vi "ABB enter motor data2.vi"(9 "Efficiency Standard":u16(ring) items=["IEC", "NEMA"], 10 "Motor Type":u16(ring) items=["Wound Induction Motor", "Induction Motor", "Synchronous Motor", "Synchronous Generator"], 11 "Efficiency Units":u16(ring) items=["METRIC", "IMPERIAL", "", "", ""]) -> (3 "entered data":string[][](array[string]))   [LabVIEW 2017]
uses:
  ABB global.vi
panel:
  in  "Specified  winding temp rise.":cluster{"Stator":dbl, "Rotor":dbl}
  out "length":i32
  in  "Explosion protection":T1 {"Gas Groups" items=["IIA", "IIB", "IIC"]; "Temp. class" items=["T3", "T2", "T1", "", ""]; "Type" items=["Exd", "EXp", "EXe", "EXn", ""]}
  in  "Synchronous Motor":T2
  in  "Specified Bearing Vibration (mm/Sec rms)":cluster{"Vibration ":dbl}={"Vibration "=1.8}
  in  "Comments":string
  in  "Vibration":T3={"Vibration(mm/sec rms)"=[[0.0, 0.0, 0.0], [0.0, 0.0, 0.0]], "Vibration µm (p-p)"=[[0.0, 0.0, 0.0], [0.0, 0.0, 0.0]], "Shaft vibration µm (p-p)"=[], "Comments"="", "Shaft Vibration"=FALSE, "DE\n\nNDE"="", "String"=""} {"Shaft vibration µm (p-p)" format="%#.2f"; "Vibration µm (p-p)" format="%#.2g"; "Vibration(mm/sec rms)" format="%#.2f"}
  in  "Axial position":T4
  in  "Exit":bool
  # "Enter Motor data 2"
  # "D"
  # "NDE"
  # "Magnetic center(mm)"
  # "-"
  # "-"
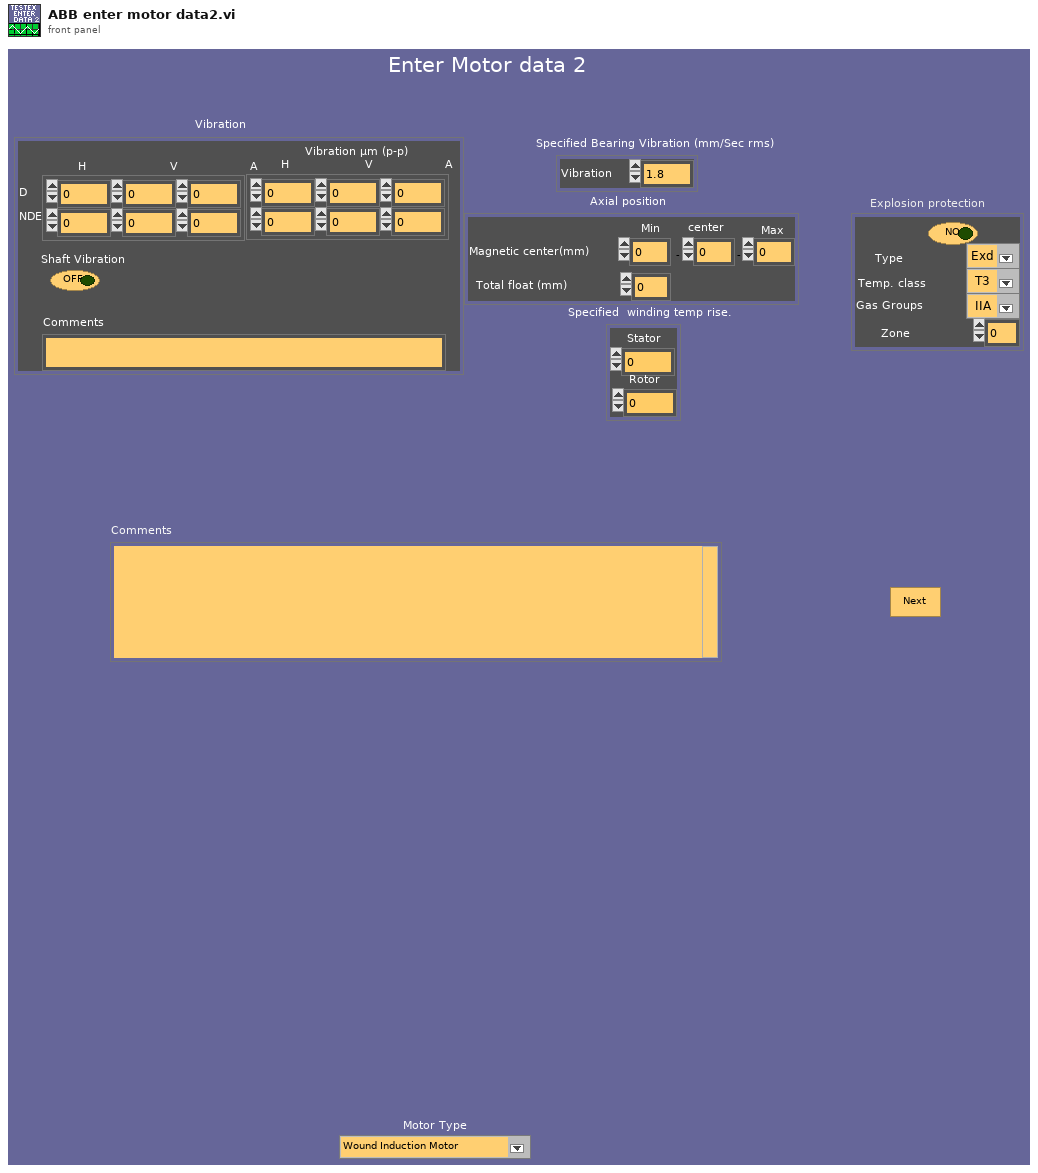
[diagram p1: front panel]
types:
  T1 = cluster{"Explosion protection":bool, "Zone":i32, "Type":u16, "Temp. class":u16, "Gas Groups":u16}
  T2 = cluster{"DC Excitation Amps":dbl, "DC Excitation Volts":dbl}
  T3 = cluster{"Vibration(mm/sec rms)":dbl[][], "Vibration µm (p-p)":dbl[][], "Shaft vibration µm (p-p)":dbl[][], "Comments":string, "Shaft Vibration":bool, "DE\n\nNDE":string, "String":string}
  T4 = cluster{"Min":dbl, " center":dbl, "Max":dbl, "Total float (mm)":dbl}
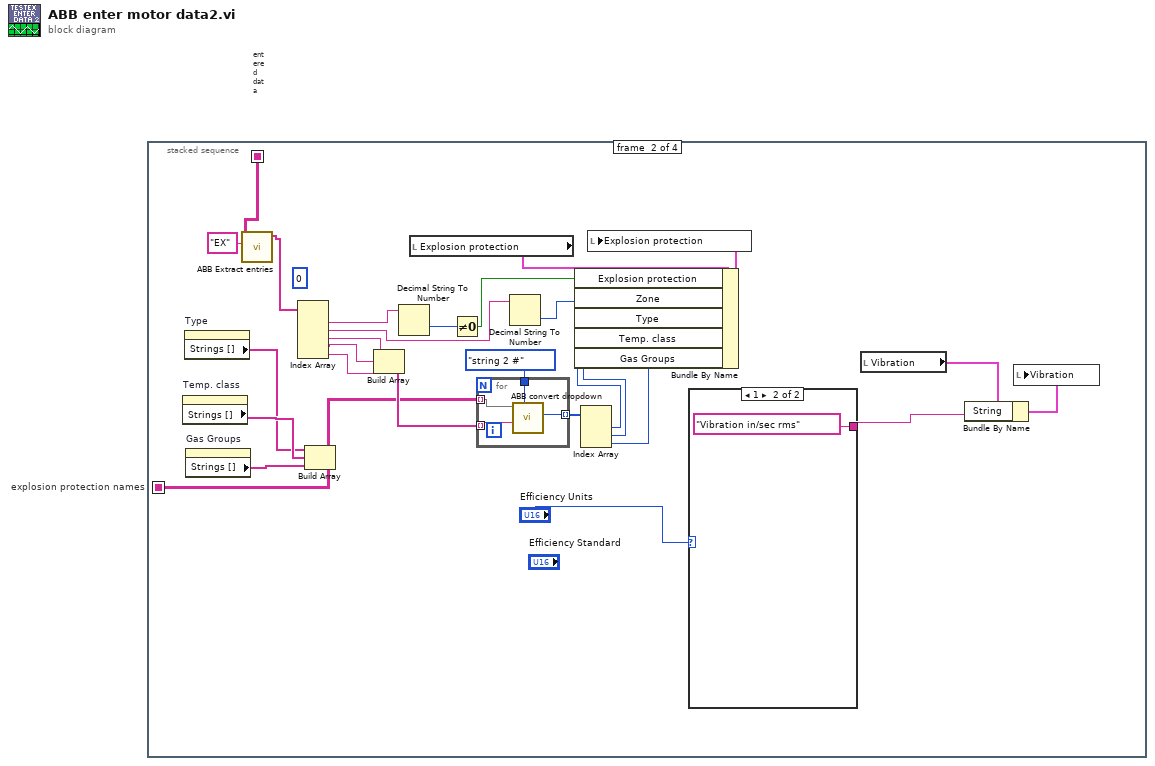
[diagram p0: block diagram]
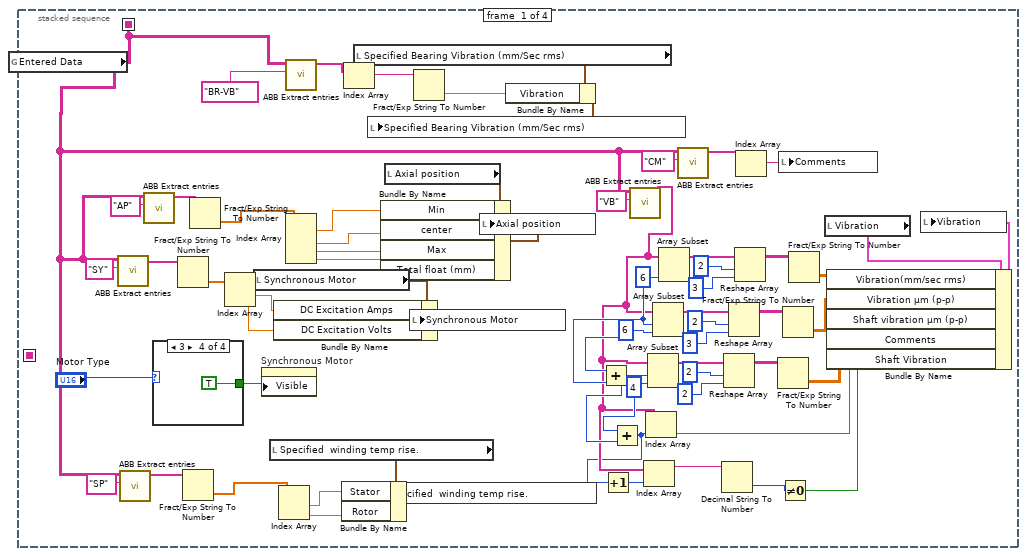
[diagram p2: hidden frame]
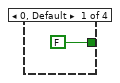
[diagram p3: hidden frame]
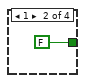
[diagram p4: hidden frame]
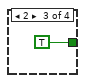
[diagram p5: hidden frame]
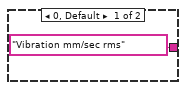
[diagram p6: hidden frame]
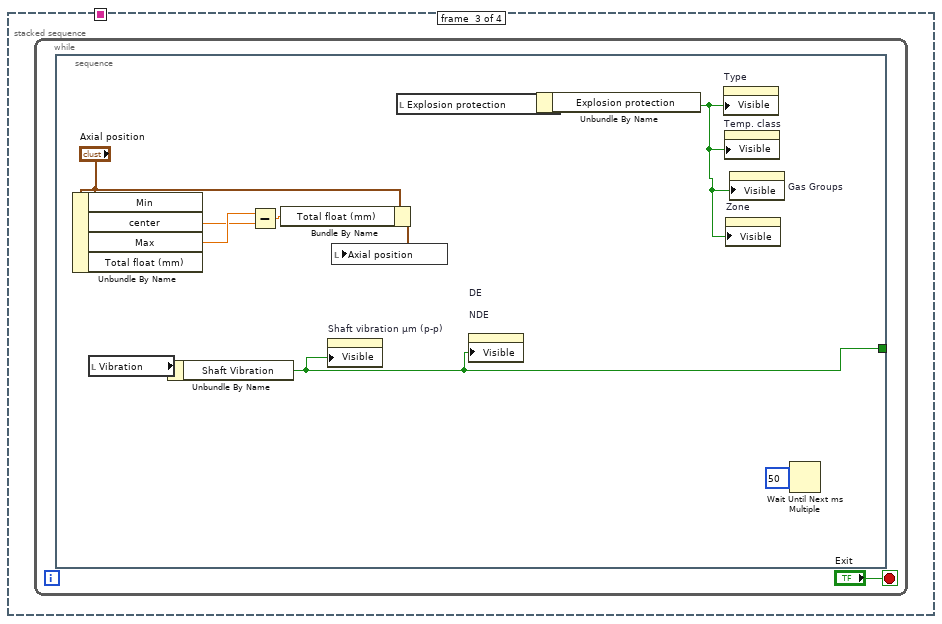
[diagram p7: hidden frame]
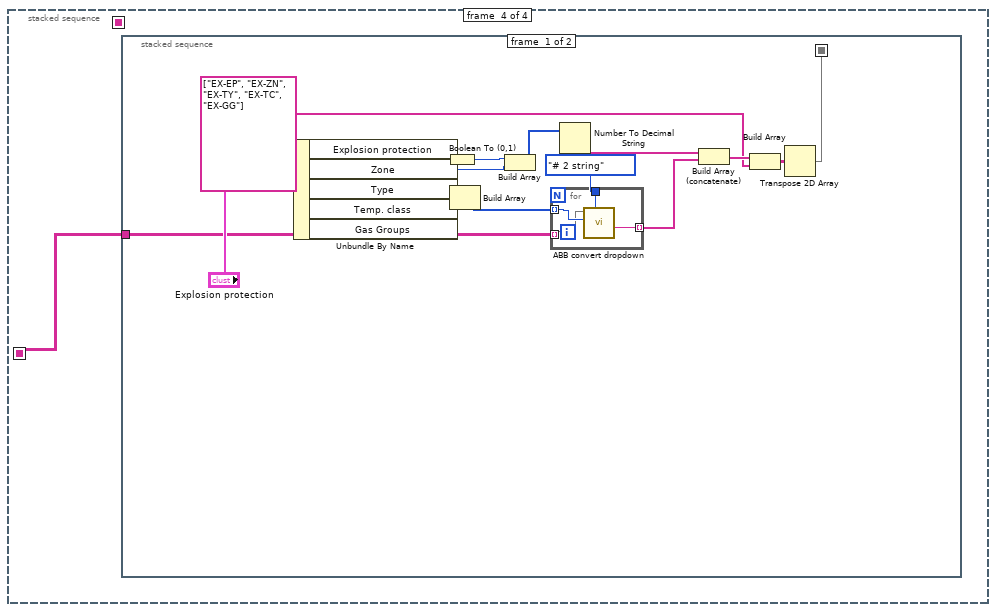
[diagram p8: hidden frame]
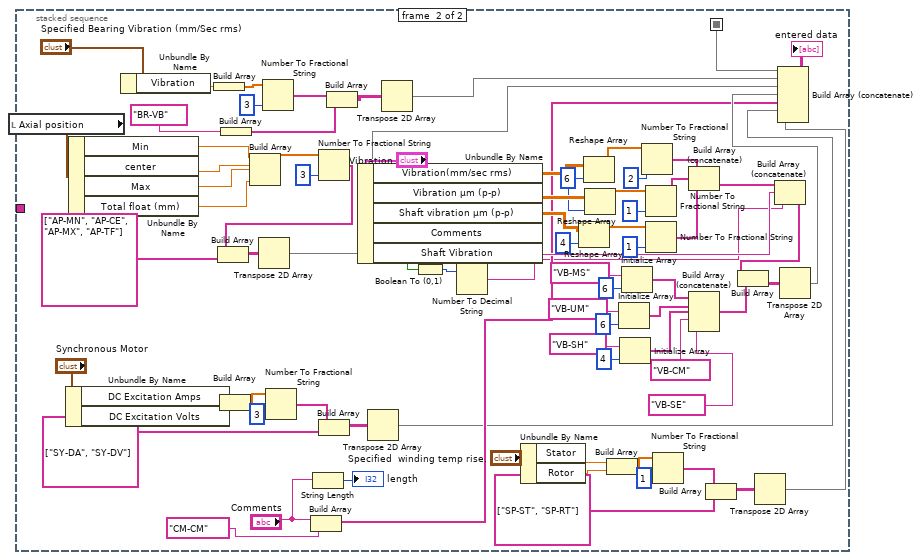
[diagram p9: hidden frame]
diagram:
  # "explosion protection names"
  # "entered data"
  n1 = stacked-sequence {
    seq-local: [w7 _ _ _] -> [_ w77 _ _]
    seq-local: [_ w73 _ _] -> [_ _ _ w113]
    frame #0 {
      w38 = 4 ("length")
      w41 = 6 ("length")
      w40 = 6 ("length")
      n2 = global read "ABB global.vi" "Entered Data"() -> (w7:string[][])
      n3 = call "ABB Extract entries.vi"("Entry ID"="SY", "Entry table in"=w7) -> ("Selected Entries"=w14:string[])  [unwired: 9 in]
      n4 = call "ABB Extract entries.vi"("Entry ID"="SP", "Entry table in"=w7) -> ("Selected Entries"=w5:string[])  [unwired: 9 in]
      n5 = call "ABB Extract entries.vi"("Entry ID"="AP", "Entry table in"=w7) -> ("Selected Entries"=w34:string[])  [unwired: 9 in]
      n6 = case shown="3" "Motor Type" {
        tunnel: [FALSE FALSE TRUE TRUE] -> w16
        frame 0, Default {
        }
        frame 1 {
        }
        frame 2 {
        }
        frame 3 {
        }
      }
      n7 = Fract/Exp String To Number(string=w14) -> (number=w13:dbl[])  [unwired: 3 in, 1 out]
      n8 = Fract/Exp String To Number(string=w5) -> (number=w6:dbl[])  [unwired: 3 in, 1 out]
      n9 = Fract/Exp String To Number(string=w34) -> (number=w62:dbl[])  [unwired: 3 in, 1 out]
      n10 = Index Array(array=w13) -> (element #1=w10:dbl, element #2=w9:dbl)  [unwired: 2 in]
      n11 = local read "Synchronous Motor"() -> (w12:T2)
      n12 = property on="Synchronous Motor" class="Clust (strict)"("Visible"=w16) -> ()  [unwired: 2 in, 2 out]
      n13 = local read "Specified  winding temp rise."() -> (w4:cluster{"Stator":dbl, "Rotor":dbl})
      n14 = Bundle By Name(cluster=w12, "DC Excitation Amps"=w10, "DC Excitation Volts"=w9) -> (w11:T2)
      n15 = Index Array(array=w6) -> (element #1=w3:dbl, element #2=w2:dbl)  [unwired: 2 in]
      n16 = call "ABB Extract entries.vi"("Entry ID"="BR-VB", "Entry table in"=w7) -> ("Selected Entries"=w28:string[])  [unwired: 9 in]
      n17 = Index Array(array=w62) -> (element #1=w61:dbl, element #2=w60:dbl, element #3=w59:dbl, element #4=w58:dbl)  [unwired: 4 in]
      n18 = Bundle By Name(cluster=w4, "Stator"=w3, "Rotor"=w2) -> (w1:cluster{"Stator":dbl, "Rotor":dbl})
      n19 = Index Array(array=w28) -> (element=w27:string)  [unwired: 1 in]
      n20 = local read "Specified Bearing Vibration (mm/Sec rms)"() -> (w26:cluster{"Vibration ":dbl})
      n21 = local write "Specified  winding temp rise."(w1) -> ()
      n22 = local read "Axial position"() -> (w64:T4)
      n23 = Bundle By Name(cluster=w64, "Min"=w61, "center"=w60, "Max"=w59, "Total float (mm)"=w58) -> (w63:T4)
      n24 = local write "Synchronous Motor"(w11) -> ()
      n25 = Fract/Exp String To Number(string=w27) -> (number=w25:dbl)  [unwired: 3 in, 1 out]
      n26 = local write "Axial position"(w63) -> ()
      n27 = Bundle By Name(cluster=w26, "Vibration"=w25) -> (w24:cluster{"Vibration ":dbl})
      n28 = local write "Specified Bearing Vibration (mm/Sec rms)"(w24) -> ()
      n29 = Add(x=w41, y=w40) -> (x+y=w37:i32)
      n30 = Add(x=w38, y=w37) -> (x+y=w22:i32)
      n31 = Increment(x=w22) -> (x+1=w21:i32)
      n32 = call "ABB Extract entries.vi"("Entry ID"="VB", "Entry table in"=w7) -> ("Selected Entries"=w23:string[])  [unwired: 9 in]
      n33 = Index Array(array=w23, index=w21) -> (element=w20:string)
      n34 = Index Array(array=w23, index=w22) -> (element=w36:string)
      n35 = Array Subset(array=w23, index=w37, length=w38) -> (w45:string[])
      n36 = Array Subset(array=w23, index=w40, length=w41) -> (w47:string[])
      n37 = Array Subset(array=w23, length=w40) -> (w57:string[])  [unwired: 1 in]
      n38 = call "ABB Extract entries.vi"("Entry ID"="CM", "Entry table in"=w7) -> ("Selected Entries"=w32:string[])  [unwired: 9 in]
      n39 = Decimal String To Number(string=w20) -> (number=w19:i32)  [unwired: 2 in, 1 out]
      n40 = Reshape Array(w45, 2 ("dimension size"), 2 ("dimension size")) -> (w42:string[][])
      n41 = Reshape Array(w47, 2 ("dimension size"), 3 ("dimension size")) -> (w50:string[][])
      n42 = Reshape Array(w57, 2 ("dimension size"), 3 ("dimension size")) -> (w53:string[][])
      n43 = Index Array(array=w32) -> (element=w31:string)  [unwired: 1 in]
      n44 = Fract/Exp String To Number(string=w42) -> (number=w39:dbl[][])  [unwired: 3 in, 1 out]
      n45 = local write "Comments"(w31) -> ()
      n46 = Not Equal To 0?(x=w19) -> (x != 0?=w18:bool)
      n47 = Fract/Exp String To Number(string=w50) -> (number=w46:dbl[][])  [unwired: 3 in, 1 out]
      n48 = Fract/Exp String To Number(string=w53) -> (number=w52:dbl[][])  [unwired: 3 in, 1 out]
      n49 = local read "Vibration"() -> (w54:T3)
      n50 = Bundle By Name(cluster=w54, "Vibration(mm/sec rms)"=w52, "Vibration µm (p-p)"=w46, "Shaft vibration µm (p-p)"=w39, "Comments"=w36, "Shaft Vibration"=w18) -> (w51:T3)
      n51 = local write "Vibration"(w51) -> ()
    }
    frame #1 {
      (unwired) 0 ("disabled index (col)")
      n52 = property on="Temp. class" class="Ring (strict)"() -> ("Strings []"=w76:string[])  [unwired: 2 in, 2 out]
      n53 = property on="Type" class="Ring (strict)"() -> ("Strings []"=w74:string[])  [unwired: 2 in, 2 out]
      n54 = property on="Gas Groups" class="Ring (strict)"() -> ("Strings []"=w75:string[])  [unwired: 2 in, 2 out]
      n55 = call "ABB Extract entries.vi"("Entry ID"="EX", "Entry table in"=w77) -> ("Selected Entries"=w78:string[])  [unwired: 9 in]
      n56 = Index Array(array=w78) -> (element #1=w95:string, element #2=w90:string, element #3=w88:string, element #4=w87:string, element #5=w86:string)  [unwired: 5 in]
      n57 = Build Array(w74, w76, w75) -> (w73:string[][])
      n58 = Build Array(w88, w87, w86) -> (w85:string[])
      n59 = Decimal String To Number(string=w95) -> (number=w94:i32)  [unwired: 2 in, 1 out]
      n60 = local read "Explosion protection"() -> (w93:T1)
      n61 = Not Equal To 0?(x=w94) -> (x != 0?=w91:bool)
      n62 = for {
        tunnel: w85 -> [w99] mode=indexing
        tunnel: w73 -> [w101] mode=indexing
        tunnel: enum16{"# 2 string", "string 2 #"}."string 2 #" ("Mode") -> [w100]
        tunnel: [w98] -> w83 mode=indexing
        n63 = call "ABB convert dropdown.vi"("Mode"=w100, "String in"=w99, "Strings"=w101) -> ("#out"=w98:i32)  [unwired: 7 in, 1 out]
      }
      n64 = Decimal String To Number(string=w90) -> (number=w89:i32)  [unwired: 2 in, 1 out]
      n65 = Index Array(array=w83) -> (element #1=w82:i32, element #2=w81:i32, element #3=w80:i32)  [unwired: 3 in]
      n66 = Bundle By Name(cluster=w93, "Explosion protection"=w91, "Zone"=w89, "Type"=w82, "Temp. class"=w81, "Gas Groups"=w80) -> (w92:T1)
      n67 = local write "Explosion protection"(w92) -> ()
      n68 = case shown="1" "Efficiency Units" {
        tunnel: ["Vibration mm/sec rms" "Vibration in/sec rms"] -> w71
        frame 0, Default {
        }
        frame 1 {
        }
      }
      n69 = local read "Vibration"() -> (w72:T3)
      n70 = Bundle By Name(cluster=w72, "String"=w71) -> (w70:T3)
      n71 = local write "Vibration"(w70) -> ()
    }
    frame #2 {
      n72 = while {
        stop <- "Exit" stop-if-true
        n73 = stacked-sequence {
          tunnel: [w105] -> _
          frame #0 {
            n74 = Unbundle By Name("Axial position") -> ("Min"=w107:dbl, "Max"=w108:dbl)  [unwired: 2 out]
            n75 = local read "Vibration"() -> (w109:T3)
            n76 = Unbundle By Name(w109) -> ("Shaft Vibration"=w105:bool)
            n77 = Subtract(x=w108, y=w107) -> (x-y=w106:dbl)
            n78 = Bundle By Name(cluster="Axial position", "Total float (mm)"=w106) -> (w110:T4)
            n79 = property on="Shaft vibration µm (p-p)" class="Arr (strict)"("Visible"=w105) -> ()  [unwired: 2 in, 2 out]
            n80 = local write "Axial position"(w110) -> ()
            n81 = local read "Explosion protection"() -> (w104:T1)
            n82 = property on="DE\n\nNDE" class="Str"("Visible"=w105) -> ()  [unwired: 2 in, 2 out]
            n83 = Unbundle By Name(w104) -> ("Explosion protection"=w103:bool)
            n84 = property on="Type" class="Ring (strict)"("Visible"=w103) -> ()  [unwired: 2 in, 2 out]
            n85 = property on="Temp. class" class="Ring (strict)"("Visible"=w103) -> ()  [unwired: 2 in, 2 out]
            n86 = property on="Zone" class="DigNum (strict)"("Visible"=w103) -> ()  [unwired: 2 in, 2 out]
            n87 = property on="Gas Groups" class="Ring (strict)"("Visible"=w103) -> ()  [unwired: 2 in, 2 out]
            n88 = Wait Until Next ms Multiple(millisecond multiple=u32 50) -> ()  [unwired: 1 out]
          }
        }
      }
    }
    frame #3 {
      n89 = stacked-sequence {
        seq-local: [w114 _] -> [_ w146]
        tunnel: w113 -> [w115 _]
        frame #0 {
          n90 = Unbundle By Name("Explosion protection") -> ("Explosion protection"=w130:bool, "Zone"=w128:i32, "Type"=w127:u16, "Temp. class"=w126:u16, "Gas Groups"=w125:u16)
          n91 = Boolean To (0,1)(Boolean=w130) -> (0, 1=w129:i16)
          n92 = Build Array(w127, w126, w125) -> (w123:u16[])
          n93 = Build Array(w129, w128) -> (w122:i32[])
          n94 = for {
            tunnel: w123 -> [w134] mode=indexing
            tunnel: w115 -> [w133] mode=indexing
            tunnel: enum16{"# 2 string", "string 2 #"}."# 2 string" ("Mode") -> [w132]
            tunnel: [w131] -> w120 mode=indexing
            n95 = call "ABB convert dropdown.vi"("Mode"=w132, "# in"=w134, "Strings"=w133) -> ("String out"=w131:string)  [unwired: 7 in, 1 out]
          }
          n96 = Number To Decimal String(number=w122) -> (decimal integer string=w121:string[])  [unwired: 1 in]
          n97 = Build Array (concatenate)(w121, w120) -> (w119:string[])
          n98 = Build Array(w119, string[] ["EX-EP", "EX-ZN", "EX-TY", "EX-TC", "EX-GG"]) -> (w118:string[][])
          n99 = Transpose 2D Array(2D array=w118) -> (transposed array=w114:string[][])
        }
        frame #1 {
          w202 = 6 ("dimension size")
          n100 = local read "Axial position"() -> (w213:T4)
          n101 = Unbundle By Name("Synchronous Motor") -> ("DC Excitation Amps"=w163:dbl, "DC Excitation Volts"=w162:dbl)
          n102 = Unbundle By Name(w213) -> ("Min"=w212:dbl, "center"=w211:dbl, "Max"=w210:dbl, "Total float (mm)"=w209:dbl)
          n103 = Unbundle By Name("Specified Bearing Vibration (mm/Sec rms)") -> ("Vibration"=w175:dbl)
          n104 = Build Array(w175) -> (w174:dbl[])
          n105 = Build Array(w163, w162) -> (w159:dbl[])
          n106 = Build Array("BR-VB") -> (w171:string[])
          n107 = Build Array(w212, w211, w210, w209) -> (w208:dbl[])
          n108 = Number To Fractional String(number=w174, precision (6)=i16 3) -> (F-format string=w173:string[])  [unwired: 2 in]
          n109 = Number To Fractional String(number=w159, precision (6)=i16 3) -> (F-format string=w160:string[])  [unwired: 2 in]
          n110 = Build Array("Comments", "CM-CM") -> (w178:string[])
          n111 = String Length(string="Comments") -> (length=→"length":i32)
          n112 = Number To Fractional String(number=w208, precision (6)=i16 3) -> (F-format string=w197:string[])  [unwired: 2 in]
          n113 = Build Array(w197, string[] ["AP-MN", "AP-CE", "AP-MX", "AP-TF"]) -> (w198:string[][])
          n114 = Transpose 2D Array(2D array=w198) -> (transposed array=w195:string[][])
          n115 = Build Array(w160, string[] ["SY-DA", "SY-DV"]) -> (w157:string[][])
          n116 = Build Array(w173, w171) -> (w170:string[][])
          n117 = Unbundle By Name("Vibration") -> ("Vibration(mm/sec rms)"=w205:dbl[][], "Vibration µm (p-p)"=w204:dbl[][], "Shaft vibration µm (p-p)"=w203:dbl[][], "Comments"=w199:string, "Shaft Vibration"=w167:bool)
          n118 = Transpose 2D Array(2D array=w157) -> (transposed array=w156:string[][])
          n119 = Transpose 2D Array(2D array=w170) -> (transposed array=w169:string[][])
          n120 = Boolean To (0,1)(Boolean=w167) -> (0, 1=w166:i16)
          n121 = Number To Decimal String(number=w166) -> (decimal integer string=w165:string)  [unwired: 1 in]
          n122 = Unbundle By Name("Specified  winding temp rise.") -> ("Stator"=w138:dbl, "Rotor"=w137:dbl)
          n123 = Reshape Array(w203, 4 ("dimension size")) -> (w149:dbl[])
          n124 = Reshape Array(w205, w202) -> (w155:dbl[])
          n125 = Reshape Array(w204, w202) -> (w153:dbl[])
          n126 = Build Array(w138, w137) -> (w141:dbl[])
          n127 = Initialize Array("VB-UM", 6 ("dimension size")) -> (w185:string[])
          n128 = Initialize Array("VB-SH", 4 ("dimension size")) -> (w186:string[])
          n129 = Initialize Array("VB-MS", 6 ("dimension size")) -> (w184:string[])
          n130 = Number To Fractional String(number=w155, precision (6)=i16 2) -> (F-format string=w154:string[])  [unwired: 2 in]
          n131 = Number To Fractional String(number=w153, precision (6)=i16 1) -> (F-format string=w152:string[])  [unwired: 2 in]
          n132 = Number To Fractional String(number=w149, precision (6)=i16 1) -> (F-format string=w148:string[])  [unwired: 2 in]
          n133 = Number To Fractional String(number=w141, precision (6)=i16 1) -> (F-format string=w140:string[])  [unwired: 2 in]
          n134 = Build Array (concatenate)(w154, w152, w148) -> (w147:string[])
          n135 = Build Array (concatenate)(w184, w185, w186, "VB-CM", "VB-SE") -> (w182:string[])
          n136 = Build Array(w140, string[] ["SP-ST", "SP-RT"]) -> (w143:string[][])
          n137 = Transpose 2D Array(2D array=w143) -> (transposed array=w135:string[][])
          n138 = Build Array (concatenate)(w147, w199, w165) -> (w183:string[])
          n139 = Build Array(w183, w182) -> (w194:string[][])
          n140 = Transpose 2D Array(2D array=w194) -> (transposed array=w181:string[][])
          n141 = Build Array (concatenate)(w146, w169, w195, w181, w178, w156, w135) -> (→"entered data":string[][])
        }
      }
    }
  }
